vi "Write Message.vi"(8 "Error In":errorcluster, 11 "Data In":T1) -> (0 "error out":errorcluster, 3 "Data Out":T1)   [LabVIEW 2014]
uses:
  Controls/TCP State Machine Data.ctl
  <vilib>/MediaMongrels Ltd/WebSockets/WebSockets/WebSockets.lvlib
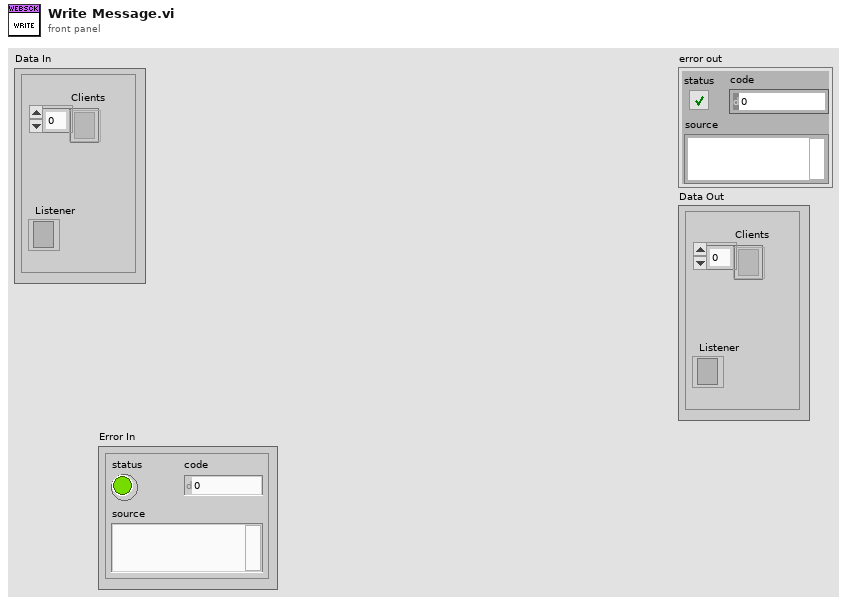
[diagram p1: front panel]
types:
  T1 = typedef "TCP State Machine Data.ctl" = cluster{"Clients":refnum<k5>[], "Listener":refnum<k5>}
  T2 = typedef "Websocket Data.ctl" = cluster{"Command":string, "Data":string}
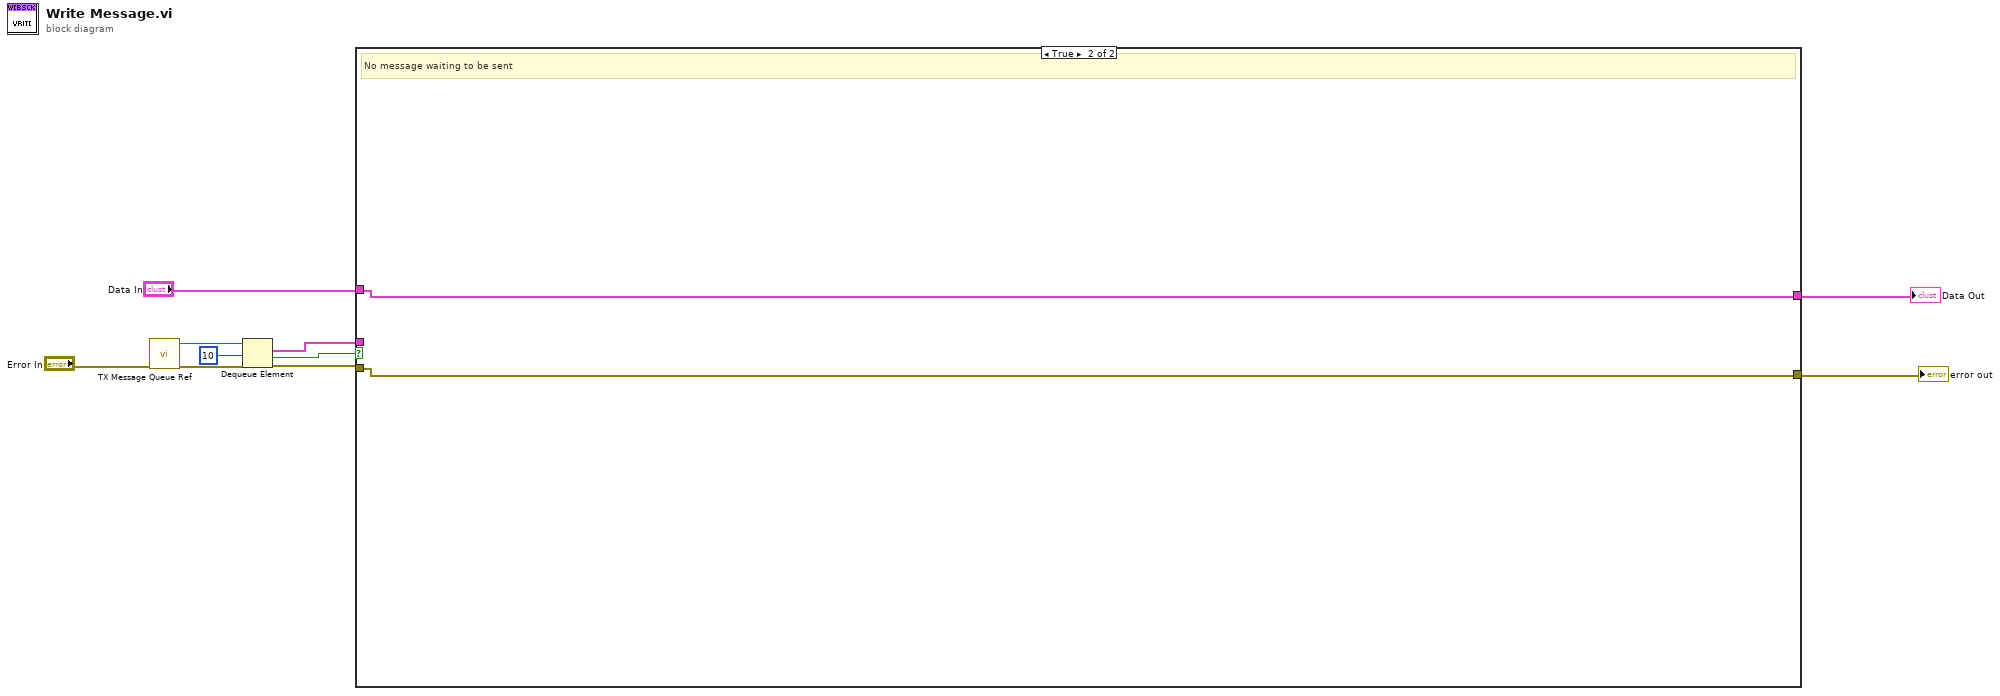
[diagram p0: block diagram]
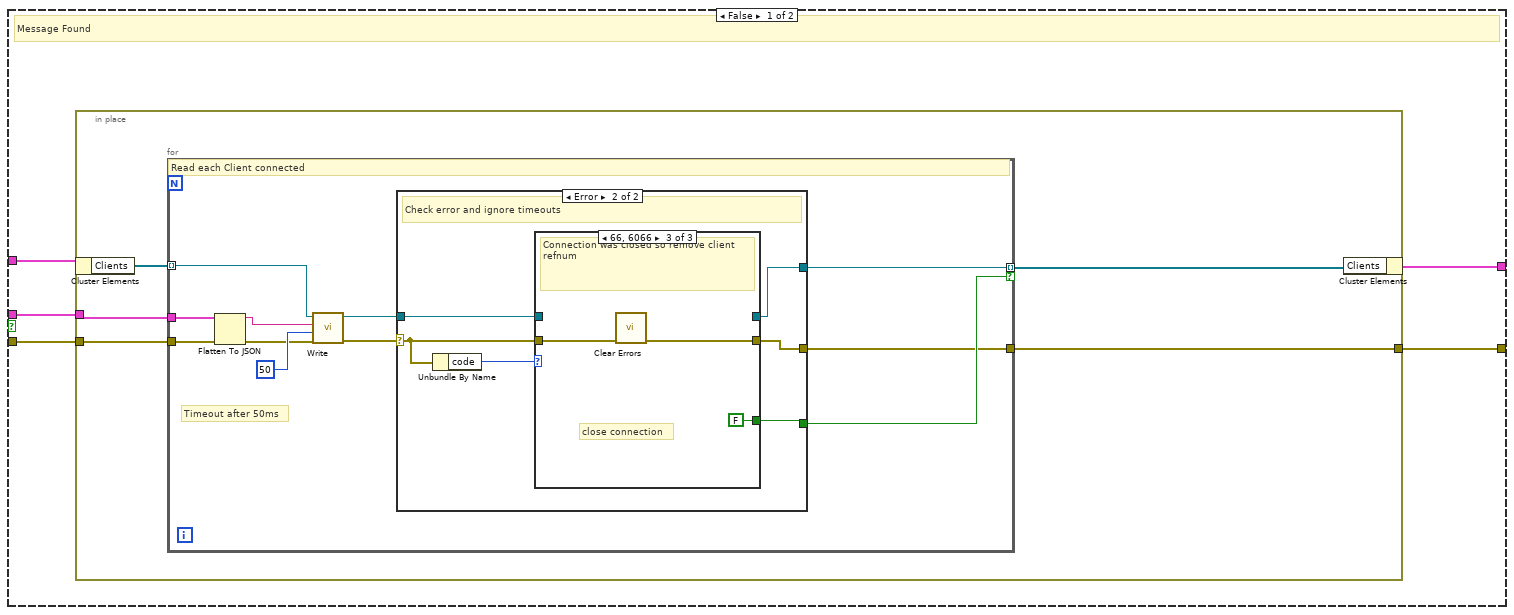
[diagram p2: hidden frame]
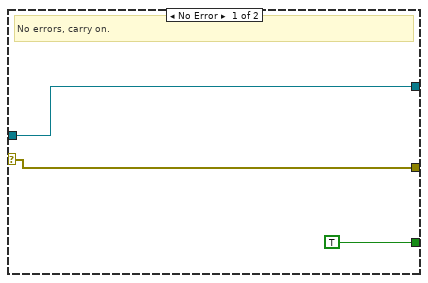
[diagram p3: hidden frame]
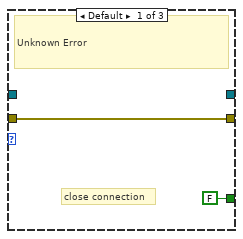
[diagram p4: hidden frame]
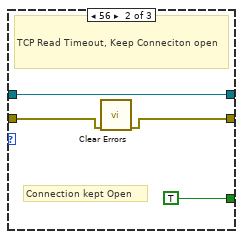
[diagram p5: hidden frame]
diagram:
  n1 = call "TX Message Queue Ref.vi"("Error In"="Error In") -> ("error out"=w4:errorcluster, "tx queue ref"=w2:refnum<queue>)  [unwired: 9 in]
  n2 = Dequeue Element(queue=w2, timeout in ms (-1)=10, error in (no error)=w4) -> (element=w5:T2, timed out?=w6:bool, error out=w7:errorcluster)  [unwired: 1 out]
  n3 = case shown="True" w6 {
    tunnel: "Data In" -> [w15 w51]
    tunnel: w7 -> [w14 w50]
    tunnel: [w13 w50] -> w9
    tunnel: [w12 w51] -> w8
    tunnel: w5 -> [w11 _]
    frame False {
      # "Message Found"
      n4 = in-place {
        in-place-border: w14 -> [w19]
        in-place-border: [w18] -> w13
        in-place-border: w11 -> [w16]
        n5 = in-place-cluster #1(w15) -> ("Clients"=w20:refnum<k5>[])
        n6 = for {
          tunnel: w20 -> [w30] mode=indexing
          tunnel: w19 -> [w25]
          tunnel: [w27] -> w17 mode=indexing if=w26
          tunnel: [w21] -> w18
          tunnel: w16 -> [w23]
          # "Timeout after 50ms"
          # "Read each Client connected"
          n7 = Flatten To JSON(anything=w23, error in (no error)=w25) -> (JSON string=w22:string, 11:w24:errorcluster)  [unwired: 1 in]
          n8 = call <vilib>:"Write.vi"("error in (no error)"=w24, "timeout ms (5000)"=50, "Data"=w22, "WebSocket Connection in"=w30) -> ("error out"=w29:errorcluster, "WebSocket Connection out"=w28:refnum<k5>)  [unwired: 6 in]
          n9 = case shown="Error" w29 {
            selector: w29 -> [w33 w38]
            tunnel: w28 -> [w32 w37]
            tunnel: [w33 w39] -> w21
            tunnel: [w32 w36] -> w27
            tunnel: [TRUE w35] -> w26
            frame No Error {
              # "No errors, carry on."
            }
            frame Error {
              # "Check error and ignore timeouts"
              n10 = Unbundle By Name(w38) -> ("code"=w40:i32)
              n11 = case shown="66, 6066" w40 {
                tunnel: [w42 w45 w49] -> w39
                tunnel: w38 -> [w42 w46 w48]
                tunnel: w37 -> [_ w44 _]
                tunnel: [_ w44 _] -> w36
                tunnel: [FALSE TRUE FALSE] -> w35
                frame Default {
                  # "close connection"
                  # "Unknown Error"
                }
                frame 56 {
                  # "Connection kept Open"
                  # "TCP Read Timeout, Keep Conneciton open"
                  n12 = call <vilib>:"Clear Errors.vi"("error in (no error)"=w46) -> ("error out"=w45:errorcluster)  [unwired: 5 in, 1 out]
                }
                frame 66, 6066 {
                  # "close connection"
                  # "Connection was closed so remove client refnum"
                  n13 = call <vilib>:"Clear Errors.vi"("error in (no error)"=w48) -> ("error out"=w49:errorcluster)  [unwired: 5 in, 1 out]
                }
              }
            }
          }
        }
        n14 = in-place-cluster #1("Clients"=w17) -> (w12:T1)
      }
    }
    frame True {
      # "No message waiting to be sent"
    }
  }
  "error out" <- w9
  "Data Out" <- w8
